vi "Set Server Key File.vi"(10 "Server Key File (.key)":path, 11 "OOP Server in":refnum<class "NW and PSD_server.lvclass">) -> (3 "OOP Server out":refnum<class "NW and PSD_server.lvclass">)   [LabVIEW 2019, in "NW and PSD_server.lvlib" / "NW and PSD_server.lvclass"]
uses:
  NW and PSD_server.lvclass
  NW and PSD_server.lvclass/NW and PSD_server.ctl
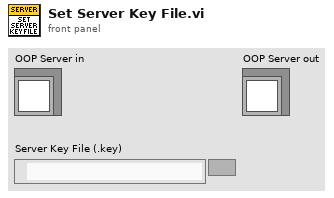
[diagram p1: front panel]
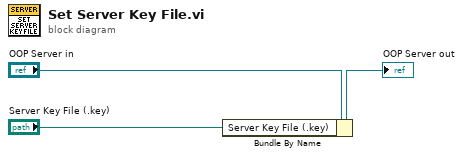
[diagram p0: block diagram]
diagram:
  n1 = Bundle By Name(cluster="OOP Server in", "Server Key File (.key)"="Server Key File (.key)") -> (→"OOP Server out":refnum<class "NW and PSD_server.lvclass">)
